vi "Encoder_PWM (6).vi"() -> ()   [LabVIEW 2019]
uses:
  <vilib>/rvi/Emulation/niFpgaGetClockAttributes.vi
  <vilib>/rvi/Emulation/niFpgaSctlEmulationGetInTimedLoop.vi
  <vilib>/rvi/Emulation/niFpgaEmulationReportErrorSimple.vi
  <vilib>/rvi/eio/common/nirviEmuTemplateMethod_errors.vi
  <vilib>/rvi/Emulation/niFpgaCriticalErrorInLSC.vi
  <vilib>/rvi/Emulation/niFpgaProcessEmulError.vi
  <vilib>/eio/EIONode/EIONode.xnode
panel:
  in  "Enable 2":bool
  in  "PWM 90% 2":i16=18000
  in  "PWM 10% 2":i16=2000
  in  "PWM Freq 2":i16=20000
  in  "Input_left":i16
  out "Enc 2":i32
  in  "Enc_Reset 2":bool
  in  "Homing Value 2":i32
  in  "Direc 2":bool
  in  "Enable":bool
  in  "PWM 90%":i16=18000
  in  "PWM 10%":i16=2000
  in  "PWM Freq":i16=20000
  in  "Input_right":i16
  in  "Direc":bool
  in  "정지":bool
  out "Enc":i32
  in  "Enc_Reset":bool
  in  "Homing Value":i32
  # "50"
  # "20"
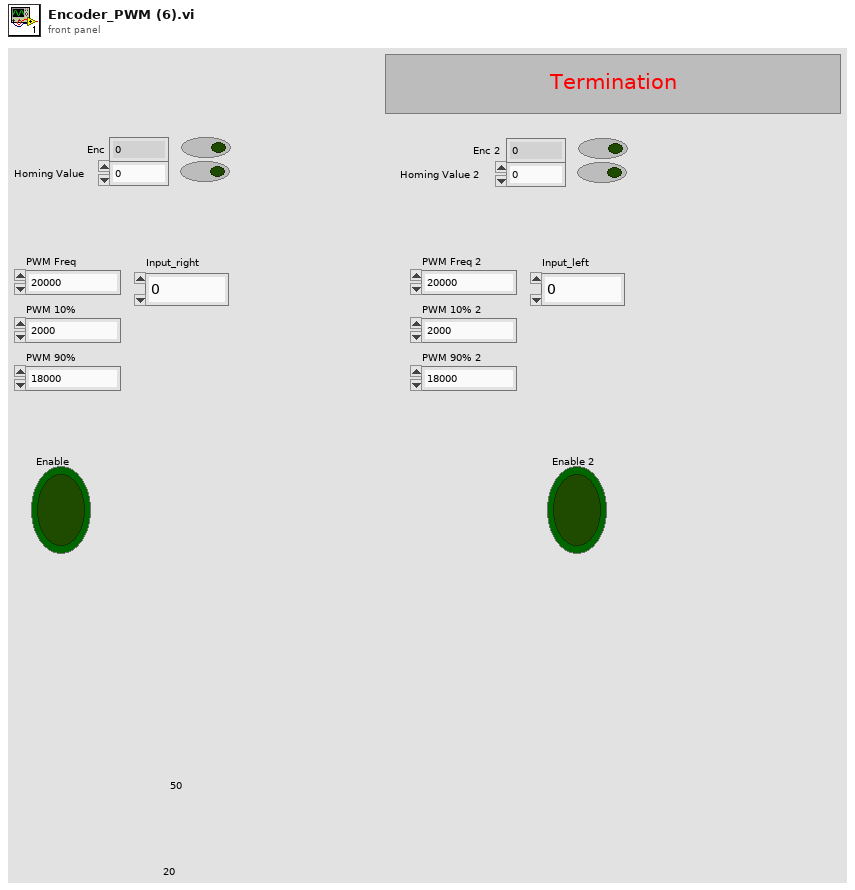
[diagram p1: front panel]
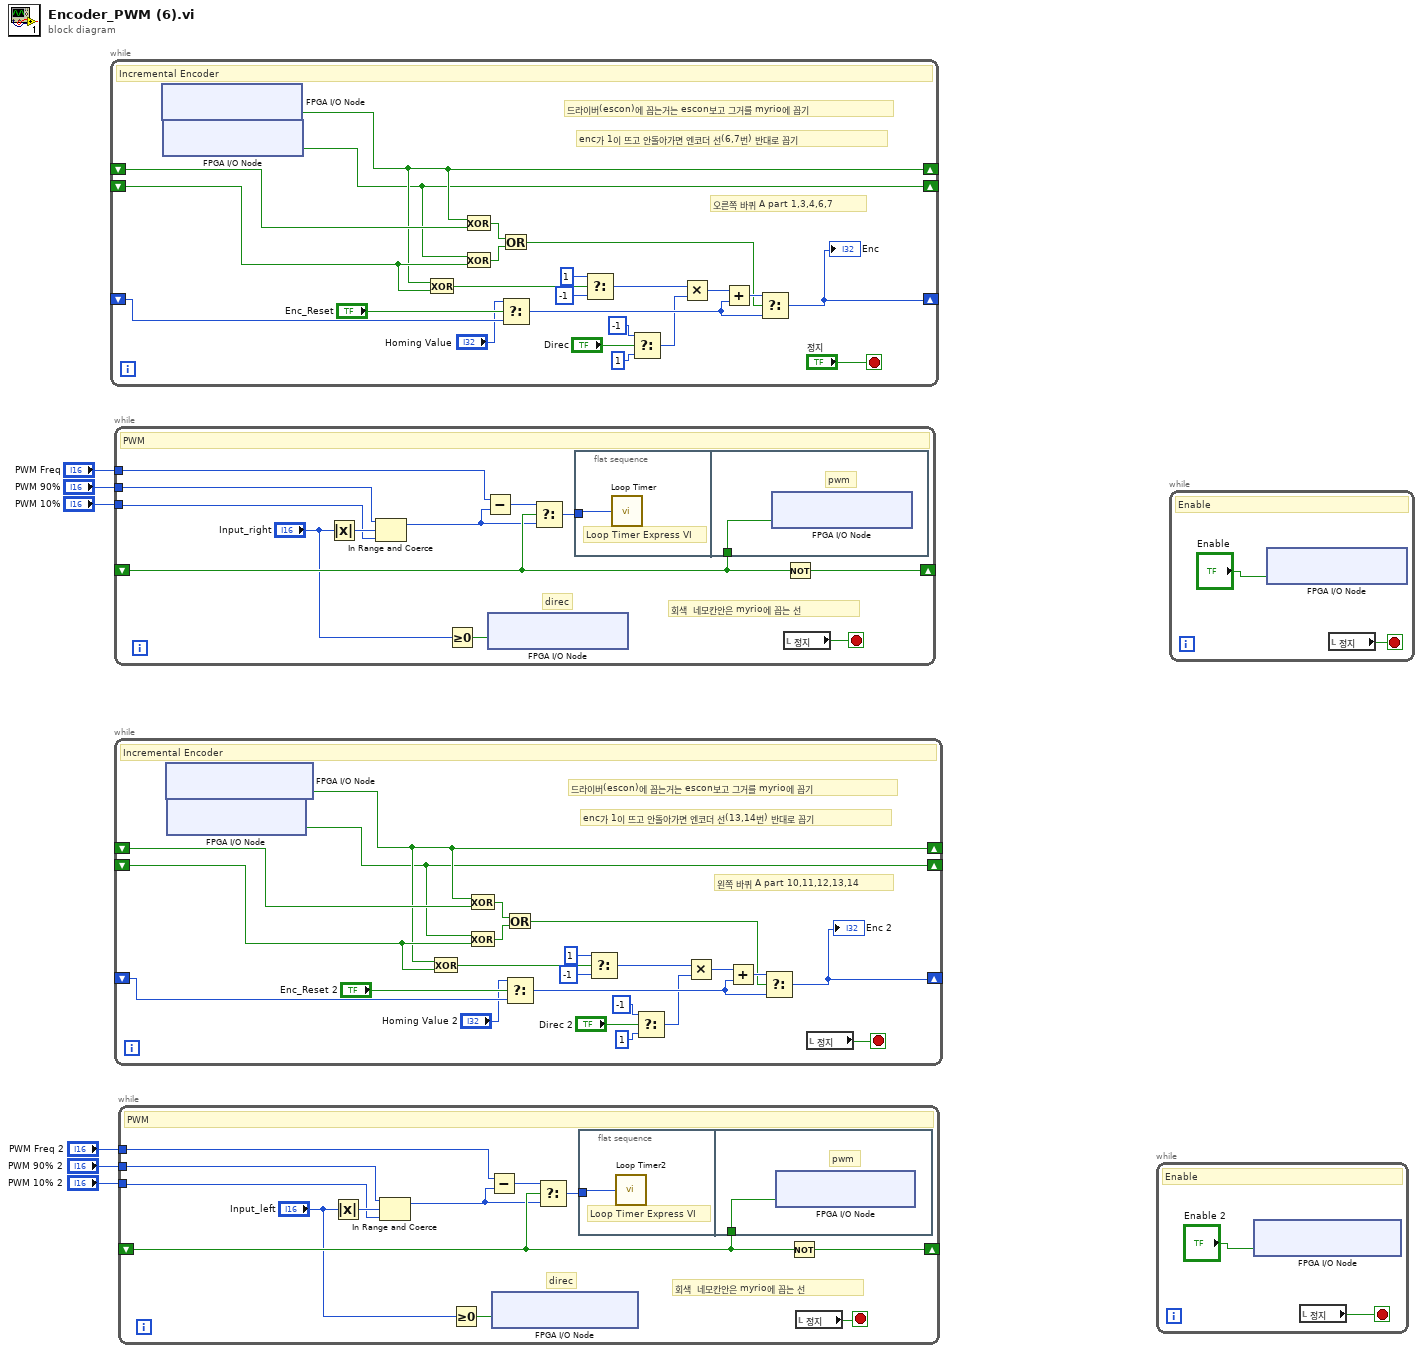
[diagram p0: block diagram]
diagram:
  n1 = while {
    shift-right: [w8] -> _
    shift-left: _ -> [w18]
    shift-right: [w7] -> _
    shift-left: _ -> [w17]
    shift-right: [w20] -> _
    shift-left: _ -> [w19]
    stop <- "정지" stop-if-true
    # "오른쪽 바퀴 A part 1,3,4,6,7"
    # "enc가 1이 뜨고 안돌아가면 엔코더 선(6,7번) 반대로 꼽기"
    # "드라이버(escon)에 꼽는거는 escon보고 그거를 myrio에 꼽기"
    # "Incremental Encoder"
    n2 = xnode "FPGA I/O Node"() -> ("ConnectorA/DIO7"=w8:bool)  [unwired: 1 in, 1 out]
    n3 = xnode "FPGA I/O Node"() -> ("ConnectorA/DIO6"=w7:bool)  [unwired: 1 in, 1 out]
    n4 = Exclusive Or(1:w17, 2:w8) -> (0:w22:bool)
    n5 = Exclusive Or(1:w18, 2:w8) -> (0:w24:bool)
    n6 = Exclusive Or(1:w17, 2:w7) -> (0:w25:bool)
    n7 = Or(x=w24, y=w25) -> (x .or. y?=w23:bool)
    n8 = Select(t="Homing Value", s="Enc_Reset", f=w19) -> (s? t:f=w28:i32)
    n9 = Select(t=i8 1 ("16 bit"), s=w22, f=i8 -1 ("16 bit")) -> (s? t:f=w11:i8)
    n10 = Select(t=i8 -1 ("16 bit"), s="Direc", f=i8 1 ("16 bit")) -> (s? t:f=w10:i8)
    n11 = Multiply(x=w11, y=w10) -> (x*y=w9:i8)
    n12 = Add(x=w9, y=w28) -> (x+y=w29:i32)
    n13 = Select(t=w29, s=w23, f=w28) -> (s? t:f=w20:i32)
    "Enc" <- w20
  }
  n14 = while "PWM Generation" {
    shift-right: [w40] -> _
    shift-left: _ -> [w38]
    tunnel: "PWM 10%" -> [w34]
    tunnel: "PWM Freq" -> [w37]
    tunnel: "PWM 90%" -> [w33]
    stop <- w31 stop-if-true
    # "회색  네모칸안은 myrio에 꼽는 선"
    # "direc"
    # "PWM"
    n15 = Absolute Value(x="Input_right") -> (abs(x)=w35:i16)
    n16 = In Range and Coerce(upper limit=w33, x=w35, lower limit=w34) -> (coerced(x)=w32:i16)  [unwired: 1 out]
    n17 = Greater Or Equal To 0?(x="Input_right") -> (x >= 0?=w30:bool)
    n18 = Subtract(x=w37, y=w32) -> (x-y=w39:i16)
    n19 = xnode "FPGA I/O Node"("ConnectorA/DIO3"=w30) -> ()  [unwired: 1 in, 1 out]
    n20 = Select(t=w39, s=w38, f=w32) -> (s? t:f=w41:i16)
    n21 = flat-sequence {
      tunnel: w41 -> [w42]
      tunnel: w38 -> [w43]
      frame #0 {
        # "Loop Timer Express VI"
        n22 = call "Loop Timer"("Count(Ticks)"=w42) -> ()  [unwired: 1 out]
      }
      frame #1 {
        # "pwm"
        n23 = xnode "FPGA I/O Node"("ConnectorA/DIO2"=w43) -> ()  [unwired: 1 in, 1 out]
      }
    }
    n24 = local read "정지"() -> (w31:bool)
    n25 = Not(x=w38) -> (.not. x?=w40:bool)
  }
  n26 = while {
    shift-right: [w46] -> _
    shift-left: _ -> [w55]
    shift-right: [w45] -> _
    shift-left: _ -> [w54]
    shift-right: [w57] -> _
    shift-left: _ -> [w56]
    stop <- w44 stop-if-true
    # "왼쪽 바퀴 A part 10,11,12,13,14"
    # "enc가 1이 뜨고 안돌아가면 엔코더 선(13,14번) 반대로 꼽기"
    # "드라이버(escon)에 꼽는거는 escon보고 그거를 myrio에 꼽기"
    # "Incremental Encoder"
    n27 = xnode "FPGA I/O Node"() -> ("ConnectorA/DIO13"=w46:bool)  [unwired: 1 in, 1 out]
    n28 = xnode "FPGA I/O Node"() -> ("ConnectorB/DIO7"=w45:bool)  [unwired: 1 in, 1 out]
    n29 = Exclusive Or(1:w54, 2:w46) -> (0:w59:bool)
    n30 = Exclusive Or(1:w55, 2:w46) -> (0:w61:bool)
    n31 = Exclusive Or(1:w54, 2:w45) -> (0:w62:bool)
    n32 = Or(x=w61, y=w62) -> (x .or. y?=w60:bool)
    n33 = Select(t="Homing Value 2", s="Enc_Reset 2", f=w56) -> (s? t:f=w65:i32)
    n34 = Select(t=i8 1 ("16 bit"), s=w59, f=i8 -1 ("16 bit")) -> (s? t:f=w49:i8)
    n35 = Select(t=i8 -1 ("16 bit"), s="Direc 2", f=i8 1 ("16 bit")) -> (s? t:f=w48:i8)
    n36 = Multiply(x=w49, y=w48) -> (x*y=w47:i8)
    n37 = Add(x=w47, y=w65) -> (x+y=w66:i32)
    n38 = Select(t=w66, s=w60, f=w65) -> (s? t:f=w57:i32)
    "Enc 2" <- w57
    n39 = local read "정지"() -> (w44:bool)
  }
  n40 = while "PWM Generation" {
    shift-right: [w77] -> _
    shift-left: _ -> [w75]
    tunnel: "PWM 10% 2" -> [w71]
    tunnel: "PWM Freq 2" -> [w74]
    tunnel: "PWM 90% 2" -> [w70]
    stop <- w67 stop-if-true
    # "회색  네모칸안은 myrio에 꼽는 선"
    # "direc"
    # "PWM"
    n41 = Absolute Value(x="Input_left") -> (abs(x)=w72:i16)
    n42 = In Range and Coerce(upper limit=w70, x=w72, lower limit=w71) -> (coerced(x)=w69:i16)  [unwired: 1 out]
    n43 = Greater Or Equal To 0?(x="Input_left") -> (x >= 0?=w68:bool)
    n44 = Subtract(x=w74, y=w69) -> (x-y=w76:i16)
    n45 = xnode "FPGA I/O Node"("ConnectorB/DIO13"=w68) -> ()  [unwired: 1 in, 1 out]
    n46 = Select(t=w76, s=w75, f=w69) -> (s? t:f=w78:i16)
    n47 = flat-sequence {
      tunnel: w78 -> [w79]
      tunnel: w75 -> [w80]
      frame #0 {
        # "Loop Timer Express VI"
        n48 = call "Loop Timer2"("Count(Ticks)"=w79) -> ()  [unwired: 1 out]
      }
      frame #1 {
        # "pwm"
        n49 = xnode "FPGA I/O Node"("ConnectorB/DIO5"=w80) -> ()  [unwired: 1 in, 1 out]
      }
    }
    n50 = Not(x=w75) -> (.not. x?=w77:bool)
    n51 = local read "정지"() -> (w67:bool)
  }
  n52 = while {
    stop <- w81 stop-if-true
    # "Enable"
    n53 = xnode "FPGA I/O Node"("ConnectorA/DIO11"="Enable 2") -> ()  [unwired: 1 in, 1 out]
    n54 = local read "정지"() -> (w81:bool)
  }
  n55 = while {
    stop <- w83 stop-if-true
    # "Enable"
    n56 = xnode "FPGA I/O Node"("ConnectorA/DIO4"="Enable") -> ()  [unwired: 1 in, 1 out]
    n57 = local read "정지"() -> (w83:bool)
  }
